vi "routine2.vi"(4 "amp3":dbl, 6 "amp1":dbl, 7 "section":i16, 9 "theta_min":dbl, 10 "theta_max":dbl, 11 "theta":dbl) -> (3 "x_d2":dbl)   [LabVIEW 2013]
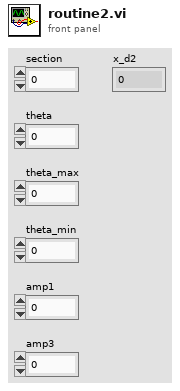
[diagram p1: front panel]
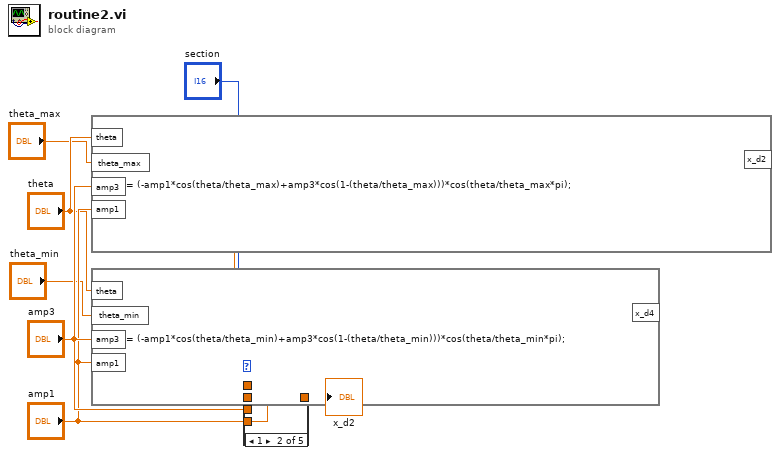
[diagram p0: block diagram]
diagram:
  n1 = formula code="x_d2 = (-amp1*cos(theta/theta_max)+amp3*cos(1-(theta/theta_max)))*cos(theta/theta_max*pi);"("theta"="theta", "theta_max"="theta_max", "amp3"="amp3", "amp1"="amp1") -> ("x_d2"=w7:dbl)
  n2 = formula code="x_d4 = (-amp1*cos(theta/theta_min)+amp3*cos(1-(theta/theta_min)))*cos(theta/theta_min*pi);"("theta"="theta", "theta_min"="theta_min", "amp3"="amp3", "amp1"="amp1") -> ("x_d4"=w9:dbl)
  n3 = case shown="1" "section" {
    tunnel: "amp1" -> [_ w10 _ _ _]
    tunnel: [_ w10 w11 w12 w13] -> w6
    tunnel: w7 -> [_ _ w11 _ _]
    tunnel: "amp3" -> [_ _ _ w12 _]
    tunnel: w9 -> [_ _ _ _ w13]
    frame 0, Default {
    }
    frame 1 {
    }
    frame 2 {
    }
    frame 3 {
    }
    frame 4 {
    }
  }
  "x_d2" <- w6
